vi "SSM.VI"(8 "error in (no error)":errorcluster caption="错误输入（无错误）", 11 "Input Data":T2) -> (0 "error out":errorcluster caption="错误输出", 3 "Output Data":T1)   [LabVIEW 2013, in "标准状态机模板.lvlib"]
uses:
  Control/Input Data.ctl
  Control/Output Data.ctl
  Control/State.ctl
  Action/Idle Enter Action.vi
  Action/Idle Action.vi
  Trans/Idle Trans.vi
  Action/Idle Exit Action.vi
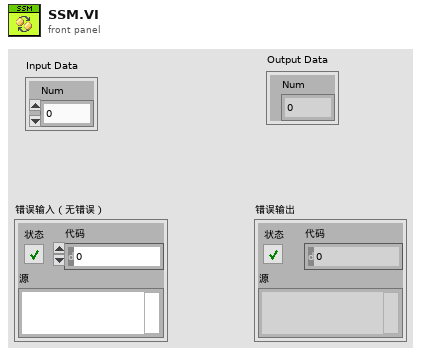
[diagram p1: front panel]
types:
  T1 = typedef "标准状态机模板.lvlib/Output Data.ctl" = cluster{"Num":dbl}
  T2 = typedef "标准状态机模板.lvlib/Input Data.ctl" = cluster{"Num":dbl}
  T3 = typedef "标准状态机模板.lvlib/State.ctl" = enum16{"Init", "Idle"}
  T4 = typedef "标准状态机模板.lvlib/SM Data.ctl" = cluster{"State":T3, "Input Data":T2, "Output Data":T1, "Internal Data":T5}
  T5 = typedef "标准状态机模板.lvlib/Internal Data.ctl" = cluster{"State Changed":bool}
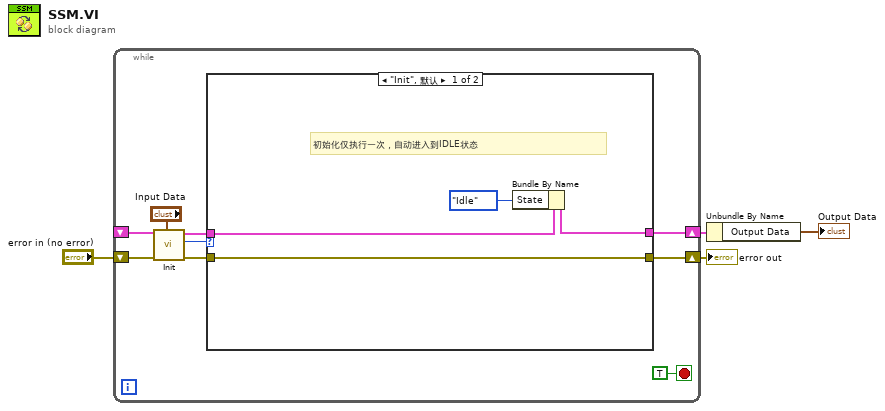
[diagram p0: block diagram]
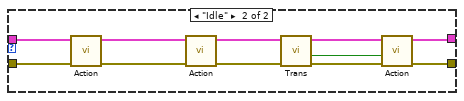
[diagram p2: hidden frame]
diagram:
  n1 = while {
    shift-right: [w7] -> w3
    shift-left: "error in (no error)" -> [w13]
    shift-right: [w10] -> w2
    shift-left: _ -> [w9]
    stop <- TRUE stop-if-true
    n2 = call "Init.vi"("Input Data"="Input Data", "error in (no error)"=w13, "SM Data In"=w9) -> ("error out"=w8:errorcluster, "State"=w12:T3, "SM Data Out"=w11:T4)  [unwired: 5 in, 1 out]
    n3 = case shown="\"Init\", 默认" w12 {
      tunnel: w11 -> [w16 w28]
      tunnel: [w15 w20] -> w10
      tunnel: w8 -> [w14 w27]
      tunnel: [w14 w22] -> w7
      frame "Init", Default {
        # "初始化仅执行一次，自动进入到IDLE状态"
        n4 = Bundle By Name(cluster=w16, "State"=State."Idle") -> (w15:T4)
      }
      frame "Idle" {
        n5 = call-poly "Action.vi"("error in (no error)"=w27, "SM Data In"=w28) -> ("error out"=w25:errorcluster, "SM Data Out"=w26:T4)  [unwired: 8 in]
        n6 = call-poly "Action.vi"("error in (no error)"=w25, "SM Data In"=w26) -> ("error out"=w24:errorcluster, "SM Data Out"=w23:T4)  [unwired: 8 in]
        n7 = call-poly "Trans.vi"("error in (no error)"=w24, "SM Data In"=w23) -> ("error out"=w19:errorcluster, "Trans Next?"=w18:bool, "SM Data Out"=w21:T4)  [unwired: 7 in]
        n8 = call-poly "Action.vi"("error in (no error)"=w19, "Exit Action"=w18, "SM Data In"=w21) -> ("error out"=w22:errorcluster, "SM Data Out"=w20:T4)  [unwired: 7 in]
      }
    }
  }
  "error out" <- w3
  n9 = Unbundle By Name(w2) -> ("Output Data"=→"Output Data":T1)
